vi "Server_Load Training Data.vi"(8 "error in":errorcluster, 11 "Name":string) -> (0 "error out":errorcluster, 3 "Training Data":T1[](array[typedef]))   [LabVIEW 2018, in "Cloud Server.lvlib"]
uses:
  Cloud Server.lvlib
  Data Def/Server_Training Data.ctl
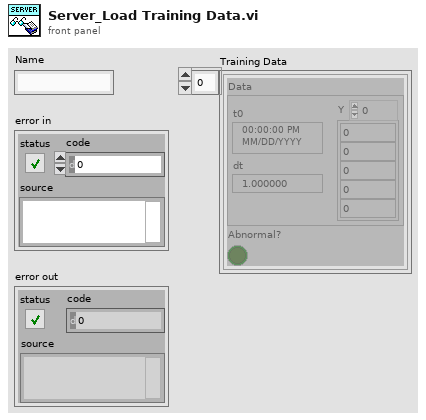
[diagram p1: front panel]
types:
  T1 = typedef "Cloud Server.lvlib/Server_Training Data.ctl" = cluster{"Data":waveform(dbl), "Abnormal?":bool}
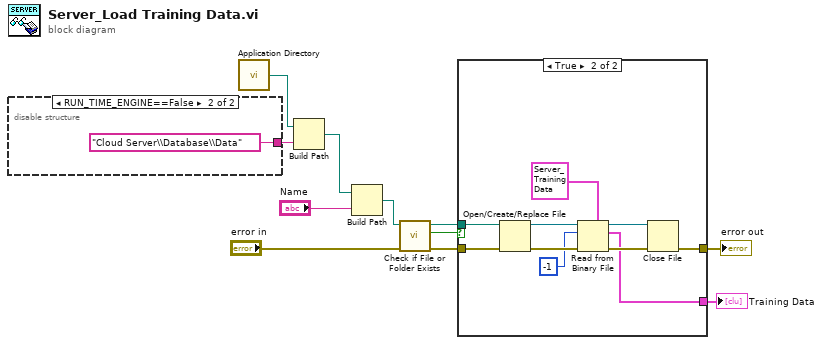
[diagram p0: block diagram]
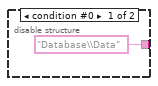
[diagram p3: hidden frame]
diagram:
  n1 = disable-structure shown="RUN_TIME_ENGINE==False" {
    disable-tunnel: ["Database\\Data" ("name or relative path") "Cloud Server\\Database\\Data" ("name or relative path")] -> w10
    frame condition #0 {
    }
    frame condition #1 (active) {
    }
  }
  n2 = call <vilib>:"Application Directory.vi"() -> ("Application Directory"=w9:path)
  n3 = Build Path(base path=w9, name or relative path=w10) -> (appended path=w8:path)
  n4 = Build Path(base path=w8, name or relative path="Name") -> (appended path=w7:path)
  n5 = call <vilib>:"Check if File or Folder Exists.vi"("error in (no error)"="error in", "path"=w7) -> ("error out"=w5:errorcluster, "file or folder exists?"=w4:bool, "dup path"=w3:path)  [unwired: 7 in]
  n6 = case shown="True" w4 {
    tunnel: w5 -> [w14 w24]
    tunnel: w3 -> [_ w23]
    tunnel: [_ w16] -> w2
    tunnel: [w14 w15] -> w1
    frame False {
    }
    frame True {
      n7 = Open/Create/Replace File(file path (use dialog)=w23, error in=w24) -> (refnum out=w21:refnum<file>, error out=w22:errorcluster)  [unwired: 4 in, 1 out]
      n8 = Read from Binary File(5:T1 {"Data"={"t0"=timestamp(0 s since 1904-01-01), "dt"=1.0, "Y"=[]}, "Abnormal?"=FALSE} ("Training Data"), 8:w22, 10:-1 ("count (1)"), 11:w21) -> (0:w19:errorcluster, 2:w16:T1[], 3:w18:refnum<file>)  [unwired: 2 in, 1 out]
      n9 = Close File(refnum=w18, error in=w19) -> (error out=w15:errorcluster)  [unwired: 1 out]
    }
  }
  "error out" <- w1
  "Training Data" <- w2
